vi "rtout_controlMode.vi"(7 "Set":bool, 8 "error in":errorcluster, 9 "mode":i32, 10 "axis in":u8, 11 "connection ID":refnum<k5>) -> (0 "error out":errorcluster, 1 "mode out":i32, 2 "axis out":i32, 3 "connection ID":refnum<k5>)   [LabVIEW 2016, in "AMC_VIs.lvlib"]
doc: "Sets or retrieves the real time output signal mode"
uses:
  AMC_VIs.lvlib
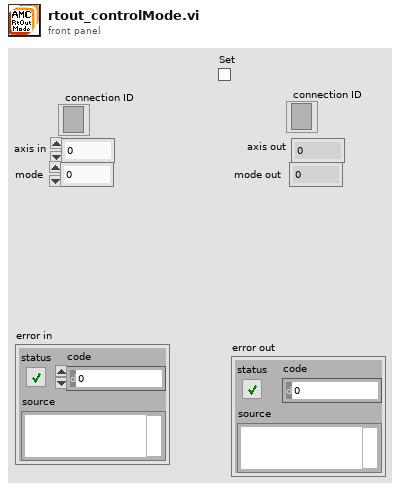
[diagram p1: front panel]
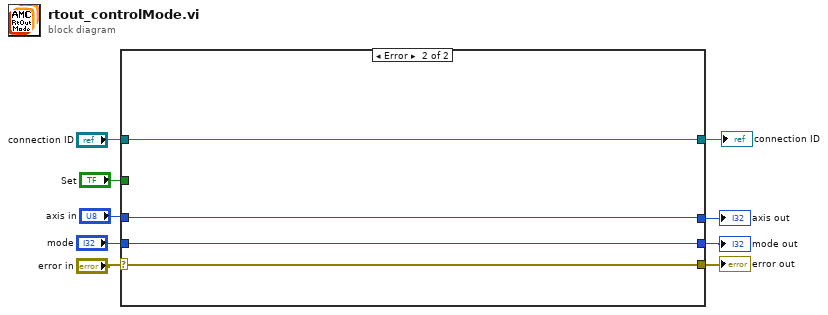
[diagram p0: block diagram]
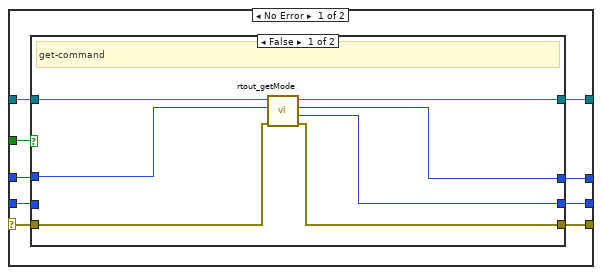
[diagram p2: hidden frame]
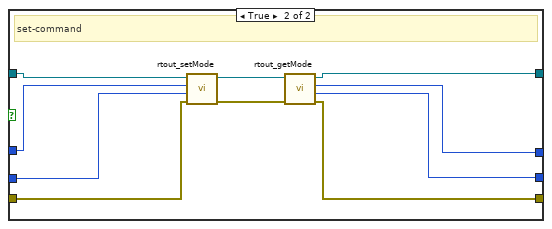
[diagram p3: hidden frame]
diagram:
  n1 = case shown="Error" "error in" {
    selector: "error in" -> [w14 w39]
    tunnel: "axis in" -> [w18 w37]
    tunnel: [w11 w39] -> w8
    tunnel: "mode" -> [w16 w38]
    tunnel: [w13 w38] -> w3
    tunnel: "Set" -> [w15 _]
    tunnel: [w12 w36] -> w6
    tunnel: "connection ID" -> [w17 w36]
    tunnel: [w10 w37] -> w1
    frame No Error {
      n2 = case shown="False" w15 {
        tunnel: w17 -> [w25 w35]
        tunnel: w18 -> [w19 w27]
        tunnel: w16 -> [_ w26]
        tunnel: w14 -> [w23 w32]
        tunnel: [w21 w29] -> w13
        tunnel: [w24 w33] -> w12
        tunnel: [w22 w30] -> w11
        tunnel: [w20 w28] -> w10
        frame False {
          # "get-command"
          n3 = call "rtout_getMode.vi"("error in"=w23, "axis"=w19, "connection ID"=w25) -> ("error out"=w22:errorcluster, "mode"=w21:i32, "axis_out"=w20:i32, "connection ID"=w24:refnum<k5>)  [unwired: 5 in]
        }
        frame True {
          # "set-command"
          n4 = call "rtout_setMode.vi"("error in"=w32, "mode"=w26, "axis"=w27, "connection ID"=w35) -> ("error out"=w31:errorcluster, "connection ID"=w34:refnum<k5>)  [unwired: 5 in, 1 out]
          n5 = call "rtout_getMode.vi"("error in"=w31, "connection ID"=w34) -> ("error out"=w30:errorcluster, "mode"=w29:i32, "axis_out"=w28:i32, "connection ID"=w33:refnum<k5>)  [unwired: 6 in]
        }
      }
    }
    frame Error {
    }
  }
  "error out" <- w8
  "axis out" <- w1
  "mode out" <- w3
  "connection ID" <- w6
